vi "chtx.vi"() -> ()   [LabVIEW 2012]
uses:
  <vilib>/addons/Modulation/Digital/General/MT Generate PSK System Parameters(M).vi
  <instrlib>/niUSRP/niUSRP Write Tx Data (CDB Cluster).vi
  <vilib>/addons/Modulation/niDMT.lvlib
panel:
  in  "BPSK System Parameters 10":T1={"Samples per Symbol"=8, "symbol map"=[], "Differential PSK"=enum."disable", "PSK type"=0} caption="BPSK System Parameters" {"PSK type" items=["normal", "shifted", "offset"]; "symbol map" format="%.3f"}
  in  "BPSK System Parameters 9":T1={"Samples per Symbol"=8, "symbol map"=[], "Differential PSK"=enum."disable", "PSK type"=0} caption="BPSK System Parameters" {"PSK type" items=["normal", "shifted", "offset"]; "symbol map" format="%.3f"}
  in  "BPSK System Parameters 8":T1={"Samples per Symbol"=8, "symbol map"=[], "Differential PSK"=enum."disable", "PSK type"=0} caption="BPSK System Parameters" {"PSK type" items=["normal", "shifted", "offset"]; "symbol map" format="%.3f"}
  in  "BPSK System Parameters 7":T1={"Samples per Symbol"=8, "symbol map"=[], "Differential PSK"=enum."disable", "PSK type"=0} caption="BPSK System Parameters" {"PSK type" items=["normal", "shifted", "offset"]; "symbol map" format="%.3f"}
  in  "BPSK System Parameters 6":T1={"Samples per Symbol"=8, "symbol map"=[], "Differential PSK"=enum."disable", "PSK type"=0} caption="BPSK System Parameters" {"PSK type" items=["normal", "shifted", "offset"]; "symbol map" format="%.3f"}
  in  "BPSK System Parameters 5":T1={"Samples per Symbol"=8, "symbol map"=[], "Differential PSK"=enum."disable", "PSK type"=0} caption="BPSK System Parameters" {"PSK type" items=["normal", "shifted", "offset"]; "symbol map" format="%.3f"}
  in  "BPSK System Parameters 4":T1={"Samples per Symbol"=8, "symbol map"=[], "Differential PSK"=enum."disable", "PSK type"=0} caption="BPSK System Parameters" {"PSK type" items=["normal", "shifted", "offset"]; "symbol map" format="%.3f"}
  out "String":string
  out "millisecond timer value":u32
  in  "millisecond multiple":u32
  in  "Tab Control":T2(tab)
  out "What is your Priority ?":string
  in  "Message Text":string="Two roads diverged in a yellow wood,\nAnd sorry I could not travel both\nAnd be one traveler, long I stood\nAnd looked down one as far as I could\nTo where it bent in the undergrowth.\n\nThen took the other, as just as fair,\nAnd having perhaps the better claim,\nBecause it was grassy and wanted wear;\nThough as for that the passing there\nHad worn them really about the same.\n\nAnd both that morning equally lay\nIn leaves no step had trodden black.\nOh, I kept the first for another day!\nYet knowing how way leads on to way,\nI doubted if I should ever come back.\n\nI shall be telling this with a sigh\nSomewhere ages and ages hence:\nTwo roads diverged in a wood, and I--\nI took the one less traveled by,\nAnd that has made all the difference.\n"
  in  "Packet Parameters":T3={"Guard Bits "=30, "Sync Bits"=20, "Message Bits"=128}
  in  "Packet Pad \n[samples]":i32=200
  in  "Blank Frame \n[samples]":i32=500
  out "Number of Packets in Message":i32=46
  in  "PN sequence order\nfor Sync Bits":i32=31 caption="PN sequence order (9)"
  in  "Packet Repeat":i32=2
  in  "Pulse Shaping Filter Parameters":T4={"Alpha"=0.5, "Filter Length"=6, "TX Filter"=enum."Root Raised Cos"} caption="Pulse Shaping Filter" {"Alpha" format="%.2f"}
  in  "Tx Parameters":T5={"Tx IQ Sampling\nRate [s/sec]"=500000.0, "Tx Frequency [Hz]"=2500000000.0, "Tx Gain [dB]"=0.0, "Tx Antenna"="TX1"} {"Tx Gain [dB]" format="%#.6p"; "Tx Frequency [Hz]" format="%#.6p"; "Tx IQ Sampling\nRate [s/sec]" format="%#.6p"}
  out "Actual Tx Parameters":T5={"Tx IQ Sampling\nRate [s/sec]"=200000.0, "Tx Frequency [Hz]"=2500000000.0, "Tx Gain [dB]"=0.0, "Tx Antenna"="TX1"} {"Tx Gain [dB]" format="%#.6p"; "Tx Frequency [Hz]" format="%#.6p"; "Tx IQ Sampling\nRate [s/sec]" format="%#.6p"}
  in  "USRP IP address":refnum<k15>="192.168.10.2"
  out "error out":errorcluster
  in  "Queue Length":i32=10
  out "Constellation Graph":T6(graph)
  in  "autoscale":bool
  out "Symbol Rate\n[symbols/sec]":dbl=25000.0 format="%#.6p"
  in  "stop":bool
  # "Guard\nBand"
  # "Sync\nSeq"
  # "Packet\nNumber"
  # "Pad\nData"
  # "Blank\nFrame"
  # "Data"
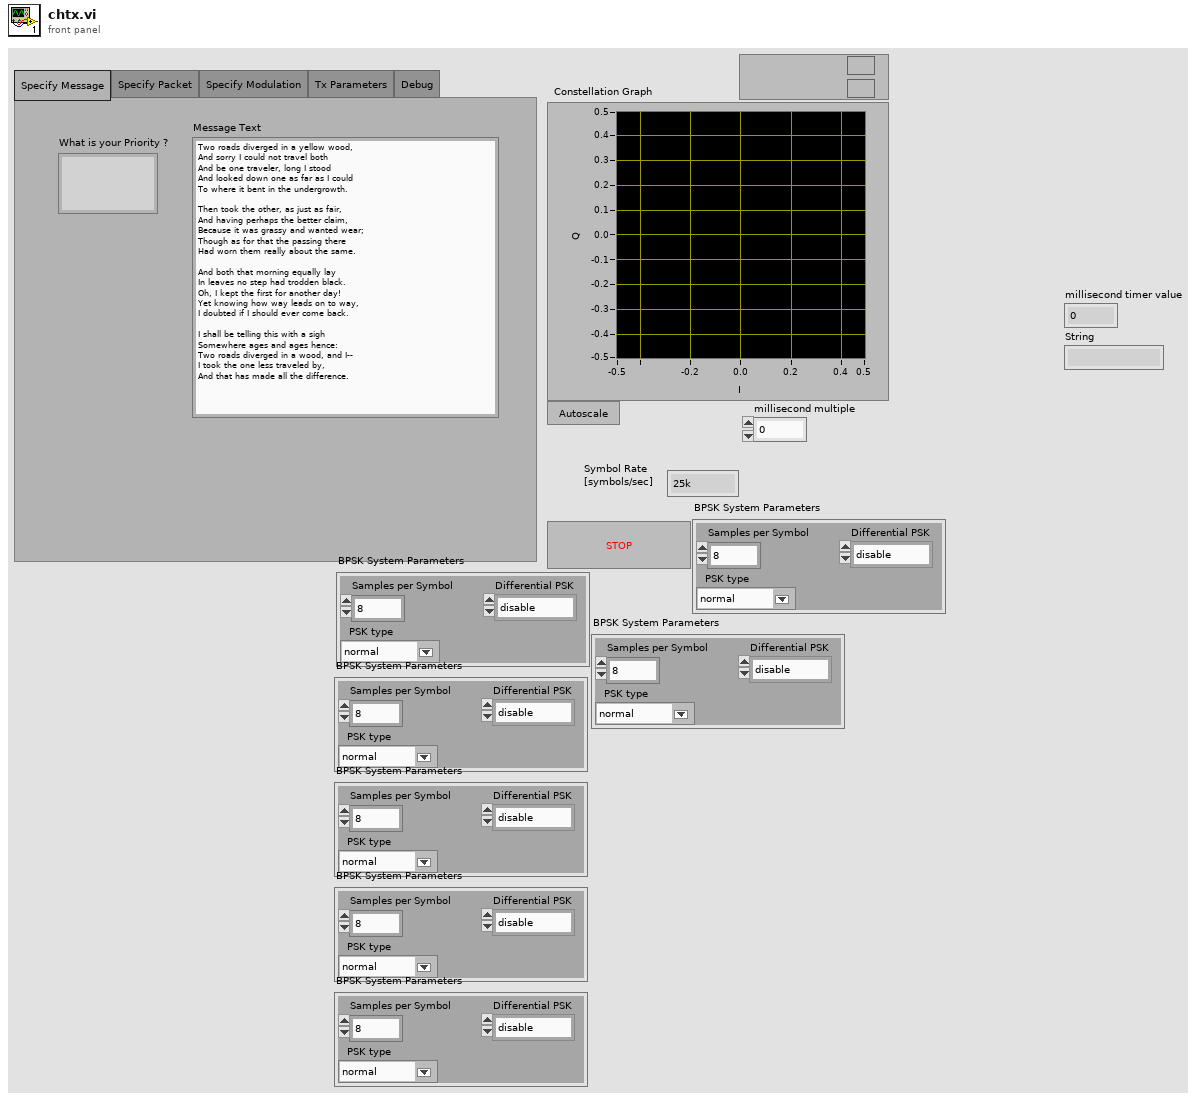
[diagram p1: front panel]
types:
  T1 = cluster{"Samples per Symbol":i32, "symbol map":cdb[], "Differential PSK":enum16{"disable", "enable"}, "PSK type":u16}
  T2 = enum32{"Specify Message", "Specify Packet", "Specify Modulation", "Tx Parameters", "Debug"}
  T3 = cluster{"Guard Bits ":i32, "Sync Bits":i32, "Message Bits":i32}
  T4 = cluster{"Alpha":dbl, "Filter Length":i32, "TX Filter":enum16{"none", "Raised Cosine", "Root Raised Cos", "Gaussian"}}
  T5 = cluster{"Tx IQ Sampling\nRate [s/sec]":dbl, "Tx Frequency [Hz]":dbl, "Tx Gain [dB]":dbl, "Tx Antenna":string}
  T6 = cluster{"Decimated Array":dbl[], "Decimated Array":dbl[]}[]
  T7 = cluster{"s? t:f":cluster{"t0":dbl, "dt":dbl, "Y":cdb[]}, i32}
  T8 = cluster{"samples per symbol (16)":i32, "symbol map":cdb[], "differential PSK":enum16{"disable", "enable"}, "PSK type":u16}
  T9 = cluster{"output complex waveform":cluster{"t0":dbl, "dt":dbl, "Y":cdb[]}, i32}
  T10 = cluster{"constellation":dbl[], "oversampled data":dbl[]}[]
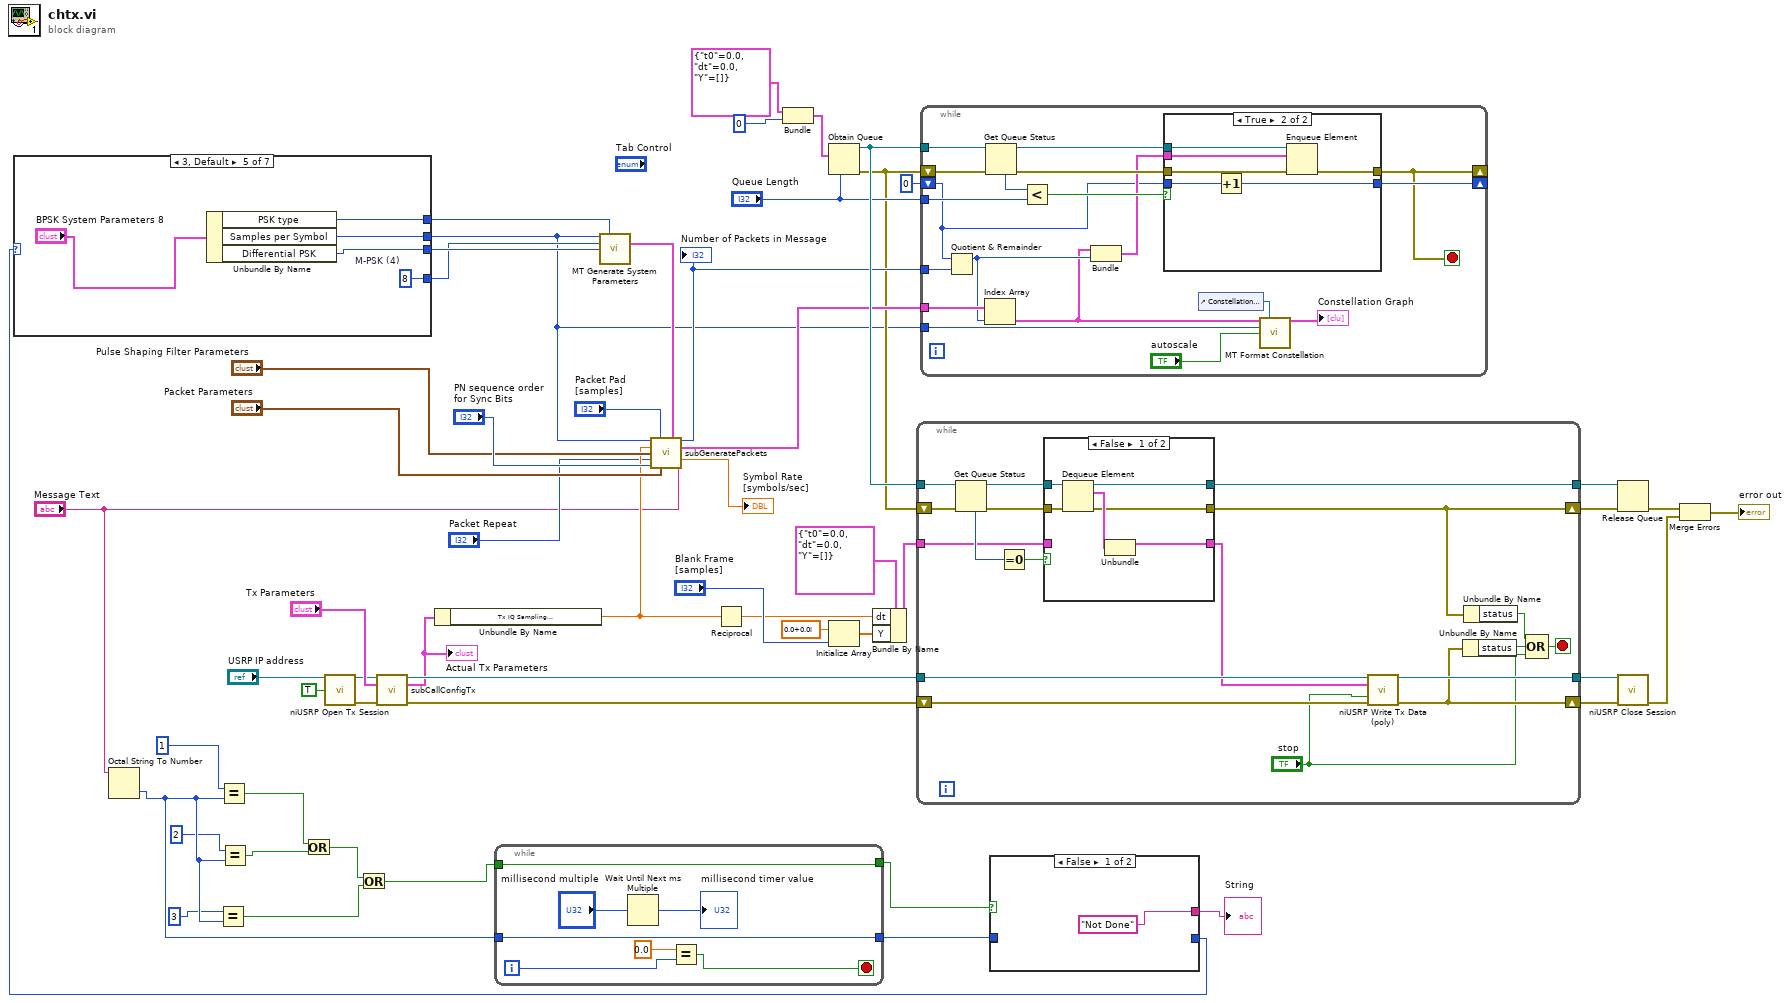
[diagram p0: block diagram]
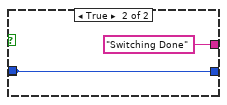
[diagram p2: hidden frame]
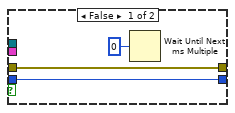
[diagram p3: hidden frame]
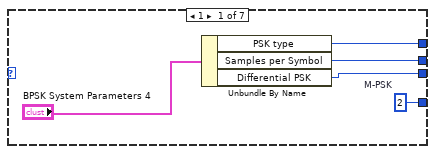
[diagram p4: hidden frame]
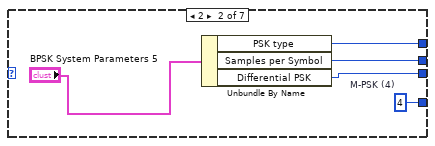
[diagram p5: hidden frame]
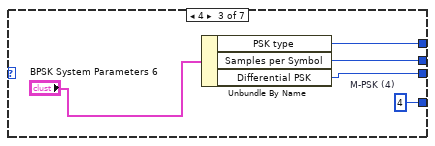
[diagram p6: hidden frame]
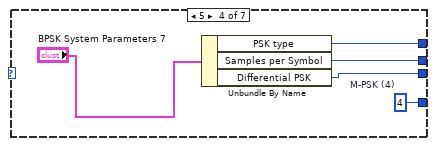
[diagram p7: hidden frame]
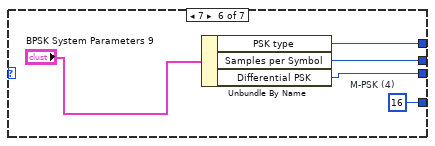
[diagram p8: hidden frame]
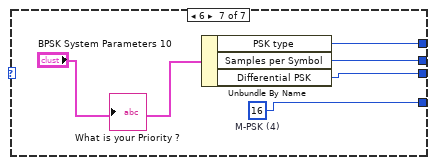
[diagram p9: hidden frame]
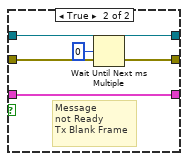
[diagram p10: hidden frame]
diagram:
  n1 = Octal String To Number(4:"Message Text") -> (0:w8:u32)  [unwired: 2 in, 1 out]
  n2 = Equal?(x=3, y=w8) -> (x = y?=w11:bool)
  n3 = Equal?(x=1, y=w8) -> (x = y?=w14:bool)
  n4 = Equal?(x=2, y=w8) -> (x = y?=w13:bool)
  n5 = Or(x=w14, y=w13) -> (x .or. y?=w12:bool)
  n6 = call <instrlib>:"niUSRP Open Tx Session.vi"("device names"="USRP IP address", "reset"=TRUE) -> ("session handle out"=w29:refnum<k15>, "error out"=w28:errorcluster)  [unwired: 12 in]
  n7 = Or(x=w12, y=w11) -> (x .or. y?=w10:bool)
  n8 = call "subCallConfigTx.vi"("session handle"=w29, "Tx Parameters"="Tx Parameters", "error in"=w28) -> ("session handle out"=w37:refnum<k15>, "Actual Tx Parameters"=w36:T5, "error out"=w42:errorcluster)  [unwired: 10 in]
  "Actual Tx Parameters" <- w36
  n9 = Unbundle By Name(w36) -> ("Tx IQ Sampling\nRate [s/sec]"=w18:dbl)
  n10 = while {
    tunnel: w10 -> [w61]
    tunnel: [w61] -> w9
    tunnel: w8 -> [w60]
    tunnel: [w60] -> w7
    i -> [w58]
    stop <- w57 stop-if-true
    n11 = Wait Until Next ms Multiple(millisecond multiple="millisecond multiple") -> (millisecond timer value=→"millisecond timer value":u32)
    n12 = Equal?(x=0.0, y=w58) -> (x = y?=w57:bool)
  }
  n13 = Reciprocal(x=w18) -> (1/x=w39:dbl)
  n14 = Bundle("s? t:f"=cluster{"t0":dbl, "dt":dbl, "Y":cdb[]} {"t0"=0.0, "dt"=0.0, "Y"=[]}, 0) -> (w47:T7)  [unwired: 1 in]
  n15 = Obtain Queue(max queue size (-1, unlimited)="Queue Length", element data type=w47) -> (queue out=w53:refnum<queue>, error out=w31:errorcluster)  [unwired: 3 in, 1 out]
  n16 = Initialize Array(cdb 0.0+0.0i ("element"), "Blank Frame \n[samples]") -> (w52:cdb[])
  n17 = Bundle By Name(cluster=cluster{"t0":dbl, "dt":dbl, "Y":cdb[]} {"t0"=0.0, "dt"=0.0, "Y"=[]} ("s? t:f"), "dt"=w39, "Y"=w52) -> (w51:cluster{"t0":dbl, "dt":dbl, "Y":cdb[]})
  n18 = while {
    tunnel: w37 -> [w72]
    shift-right: [w69] -> w41
    shift-left: w42 -> [w73]
    tunnel: w53 -> [w81]
    tunnel: w51 -> [w78]
    tunnel: [w77] -> w50
    tunnel: [w71] -> w40
    shift-right: [w66] -> w49
    shift-left: w31 -> [w74]
    stop <- w68 stop-if-true
    n19 = Get Queue Status(queue=w81, error in (no error)=w74) -> (queue out=w76:refnum<queue>, error out=w75:errorcluster, # elements in queue=w80:i32)  [unwired: 1 in, 5 out]
    n20 = Equal To 0?(x=w80) -> (x = 0?=w79:bool)
    n21 = case shown="False" w79 {
      tunnel: w78 -> [_ w91]
      tunnel: [w83 w91] -> w64
      tunnel: [w87 w89] -> w77
      tunnel: [w82 w90] -> w66
      tunnel: w76 -> [w86 w89]
      tunnel: w75 -> [w85 w90]
      frame False {
        n22 = Dequeue Element(queue=w86, error in (no error)=w85) -> (queue out=w87:refnum<queue>, element=w84:T7, error out=w82:errorcluster)  [unwired: 1 in, 1 out]
        n23 = Unbundle(w84) -> ("s? t:f"=w83:cluster{"t0":dbl, "dt":dbl, "Y":cdb[]})  [unwired: 1 out]
      }
      frame True {
        # "Message\nnot Ready\nTx Blank Frame"
        n24 = Wait Until Next ms Multiple(millisecond multiple=u32 0) -> ()  [unwired: 1 out]
      }
    }
    n25 = call-poly <instrlib>:"niUSRP Write Tx Data (poly).vi"("session handle"=w72, "data"=w64, "end of data?"="stop", "error in (no error)"=w73) -> ("session handle out"=w71:refnum<k15>, "error out"=w69:errorcluster)  [unwired: 10 in]
    n26 = Unbundle By Name(w69) -> ("status"=w70:bool)
    n27 = Unbundle By Name(w66) -> ("status"=w65:bool)
    n28 = Compound Arithmetic op=OR(w65, w70, "stop") -> (w68:bool)
  }
  n29 = case shown="False" w9 {
    tunnel: [_ w93] -> _
    tunnel: w7 -> [_ w93]
    tunnel: ["Not Done" "Switching Done"] -> w6
    tunnel: [_ w93] -> w1
    frame False {
    }
    frame True {
    }
  }
  "String" <- w6
  n30 = case shown="3, Default" w1 {
    tunnel: [w96 w101 w108 w113 w118 w124 w127] -> w17
    tunnel: [w97 w102 w107 w112 w117 w123 w128] -> w56
    tunnel: [w99 w104 w109 w114 w116 w122 w125] -> w38
    tunnel: [w98 w103 w106 w111 w119 w121 w129] -> w25
    frame 1 {
      w99 = 2  # M-PSK
      n31 = Unbundle By Name("BPSK System Parameters 4") -> ("PSK type"=w98:u16, "Samples per Symbol"=w96:i32, "Differential PSK"=w97:enum16{"disable", "enable"})
    }
    frame 2 {
      w104 = 4  # M-PSK (4)
      n32 = Unbundle By Name("BPSK System Parameters 5") -> ("PSK type"=w103:u16, "Samples per Symbol"=w101:i32, "Differential PSK"=w102:enum16{"disable", "enable"})
    }
    frame 4 {
      w109 = 4  # M-PSK (4)
      n33 = Unbundle By Name("BPSK System Parameters 6") -> ("PSK type"=w106:u16, "Samples per Symbol"=w108:i32, "Differential PSK"=w107:enum16{"disable", "enable"})
    }
    frame 5 {
      w114 = 4  # M-PSK (4)
      n34 = Unbundle By Name("BPSK System Parameters 7") -> ("PSK type"=w111:u16, "Samples per Symbol"=w113:i32, "Differential PSK"=w112:enum16{"disable", "enable"})
    }
    frame 3, Default {
      w116 = 8  # M-PSK (4)
      n35 = Unbundle By Name("BPSK System Parameters 8") -> ("PSK type"=w119:u16, "Samples per Symbol"=w118:i32, "Differential PSK"=w117:enum16{"disable", "enable"})
    }
    frame 7 {
      w122 = 16  # M-PSK (4)
      n36 = Unbundle By Name("BPSK System Parameters 9") -> ("PSK type"=w121:u16, "Samples per Symbol"=w124:i32, "Differential PSK"=w123:enum16{"disable", "enable"})
    }
    frame 6 {
      w125 = 16  # M-PSK (4)
      n37 = Unbundle By Name("BPSK System Parameters 10") -> ("PSK type"=w129:u16, "Samples per Symbol"=w127:i32, "Differential PSK"=w128:enum16{"disable", "enable"})
    }
  }
  n38 = call-poly <vilib>:"MT Generate System Parameters.vi"("samples per symbol (16)"=w17, "PSK type"=w25, "M-PSK (4)"=w38, "differential PSK"=w56) -> ("PSK system parameters"=w26:T8)  [unwired: 9 in, 2 out]
  n39 = call "subGeneratePackets.vi"("Samples per Symbol"=w17, "Packet Pad \n[samples]"="Packet Pad \n[samples]", "PSK system parameters"=w26, "Tx IQ Sampling\nRate [s/sec]"=w18, "Pulse Shaping Filter Parameters"="Pulse Shaping Filter Parameters", "Packet Repeat"="Packet Repeat", "PN sequence order\nfor Sync Bits"="PN sequence order\nfor Sync Bits", "Packet Parameters"="Packet Parameters", "Message Text"="Message Text") -> ("Number of Packets"=w35:i32, "Packets"=w44:cluster{"t0":dbl, "dt":dbl, "Y":cdb[]}[], "Symbol Rate"=→"Symbol Rate\n[symbols/sec]":dbl)  [unwired: 4 in]
  "Number of Packets in Message" <- w35
  n40 = while {
    tunnel: w53 -> [w148]
    shift-right: [w141] -> _
    shift-left: 0 -> [w137]
    tunnel: w44 -> [w138]
    tunnel: "Queue Length" -> [w140]
    tunnel: w35 -> [w139]
    shift-right: [w135] -> _
    shift-left: w31 -> [w143]
    tunnel: w17 -> [w132]
    stop <- w135 stop-if-true
    n41 = Quotient & Remainder(x=w137, y=w139) -> (x-y*floor(x/y)=w136:i32)  [unwired: 1 out]
    n42 = Index Array(array=w138, index=w136) -> (element=w130:cluster{"t0":dbl, "dt":dbl, "Y":cdb[]})
    n43 = Get Queue Status(queue=w148, error in (no error)=w143) -> (queue out=w147:refnum<queue>, error out=w144:errorcluster, # elements in queue=w146:i32)  [unwired: 1 in, 5 out]
    n44 = Less?(x=w146, y=w140) -> (x < y?=w145:bool)
    n45 = Bundle("output complex waveform"=w130, w136) -> (w142:T9)  [unwired: 1 in]
    n46 = case shown="True" w145 {
      tunnel: w144 -> [w149 w157]
      tunnel: w147 -> [_ w156]
      tunnel: [w149 w155] -> w135
      tunnel: w142 -> [_ w154]
      tunnel: w137 -> [w151 w153]
      tunnel: [w151 w152] -> w141
      frame False {
        n47 = Wait Until Next ms Multiple(millisecond multiple=u32 0) -> ()  [unwired: 1 out]
      }
      frame True {
        n48 = Increment(x=w153) -> (x+1=w152:i32)
        n49 = Enqueue Element(queue=w156, element=w154, error in (no error)=w157) -> (error out=w155:errorcluster)  [unwired: 1 in, 2 out]
      }
    }
    n50 = control-ref of="Constellation Graph"() -> (w133:refnum<vi>)
    n51 = call <vilib>:"MT Format Constellation.vi"("waveform"=w130, "constellation reference"=w133, "samples per symbol"=w132, "autoscale"="autoscale") -> ("constellation graph"=→"Constellation Graph":T10)  [unwired: 1 in, 10 out]
  }
  n52 = Release Queue(queue=w50, error in (no error)=w49) -> (error out=w24:errorcluster)  [unwired: 3 out]
  n53 = call <instrlib>:"niUSRP Close Session.vi"("session handle"=w40, "error in (no error)"=w41) -> ("error out"=w23:errorcluster)  [unwired: 13 in]
  n54 = Merge Errors(w24, w23) -> (→"error out":errorcluster)
